vi "main.vi"() -> ()   [LabVIEW 2015]
panel:
  out "selected path":path caption="선택된 경로"
  in  "Del":bool
  in  "정지 버튼":bool
  out "원소의 인덱스":i32
  out "Right 3":cluster{"Max":u32, "Min":u32, "Delta":u32}
  out "Right 2":cluster{"Max":u32, "Min":u32, "Delta":u32}
  out "Right 1":cluster{"Max":u32, "Min":u32, "Delta":u32}
  out "Left 3":cluster{"Max":u32, "Min":u32, "Delta":u32}
  out "Left 2":cluster{"Max":u32, "Min":u32, "Delta":u32}
  out "Left 1":cluster{"Max":u32, "Min":u32, "Delta":u32}
  out "XY 그래프":cluster{"Time(s)":dbl[], "calculation":u32[]}[](graph)
  # "Chart Name"
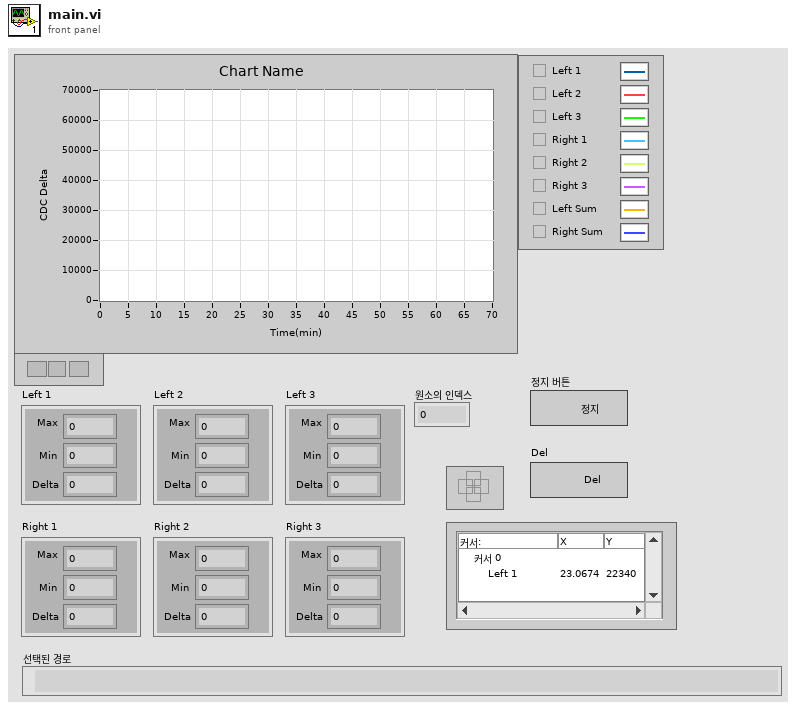
[diagram p1: front panel]
types:
  T1 = cluster{"raw data":u32[], "max":u32, "min":u32, "delta":u32, "calculation":u32[]}
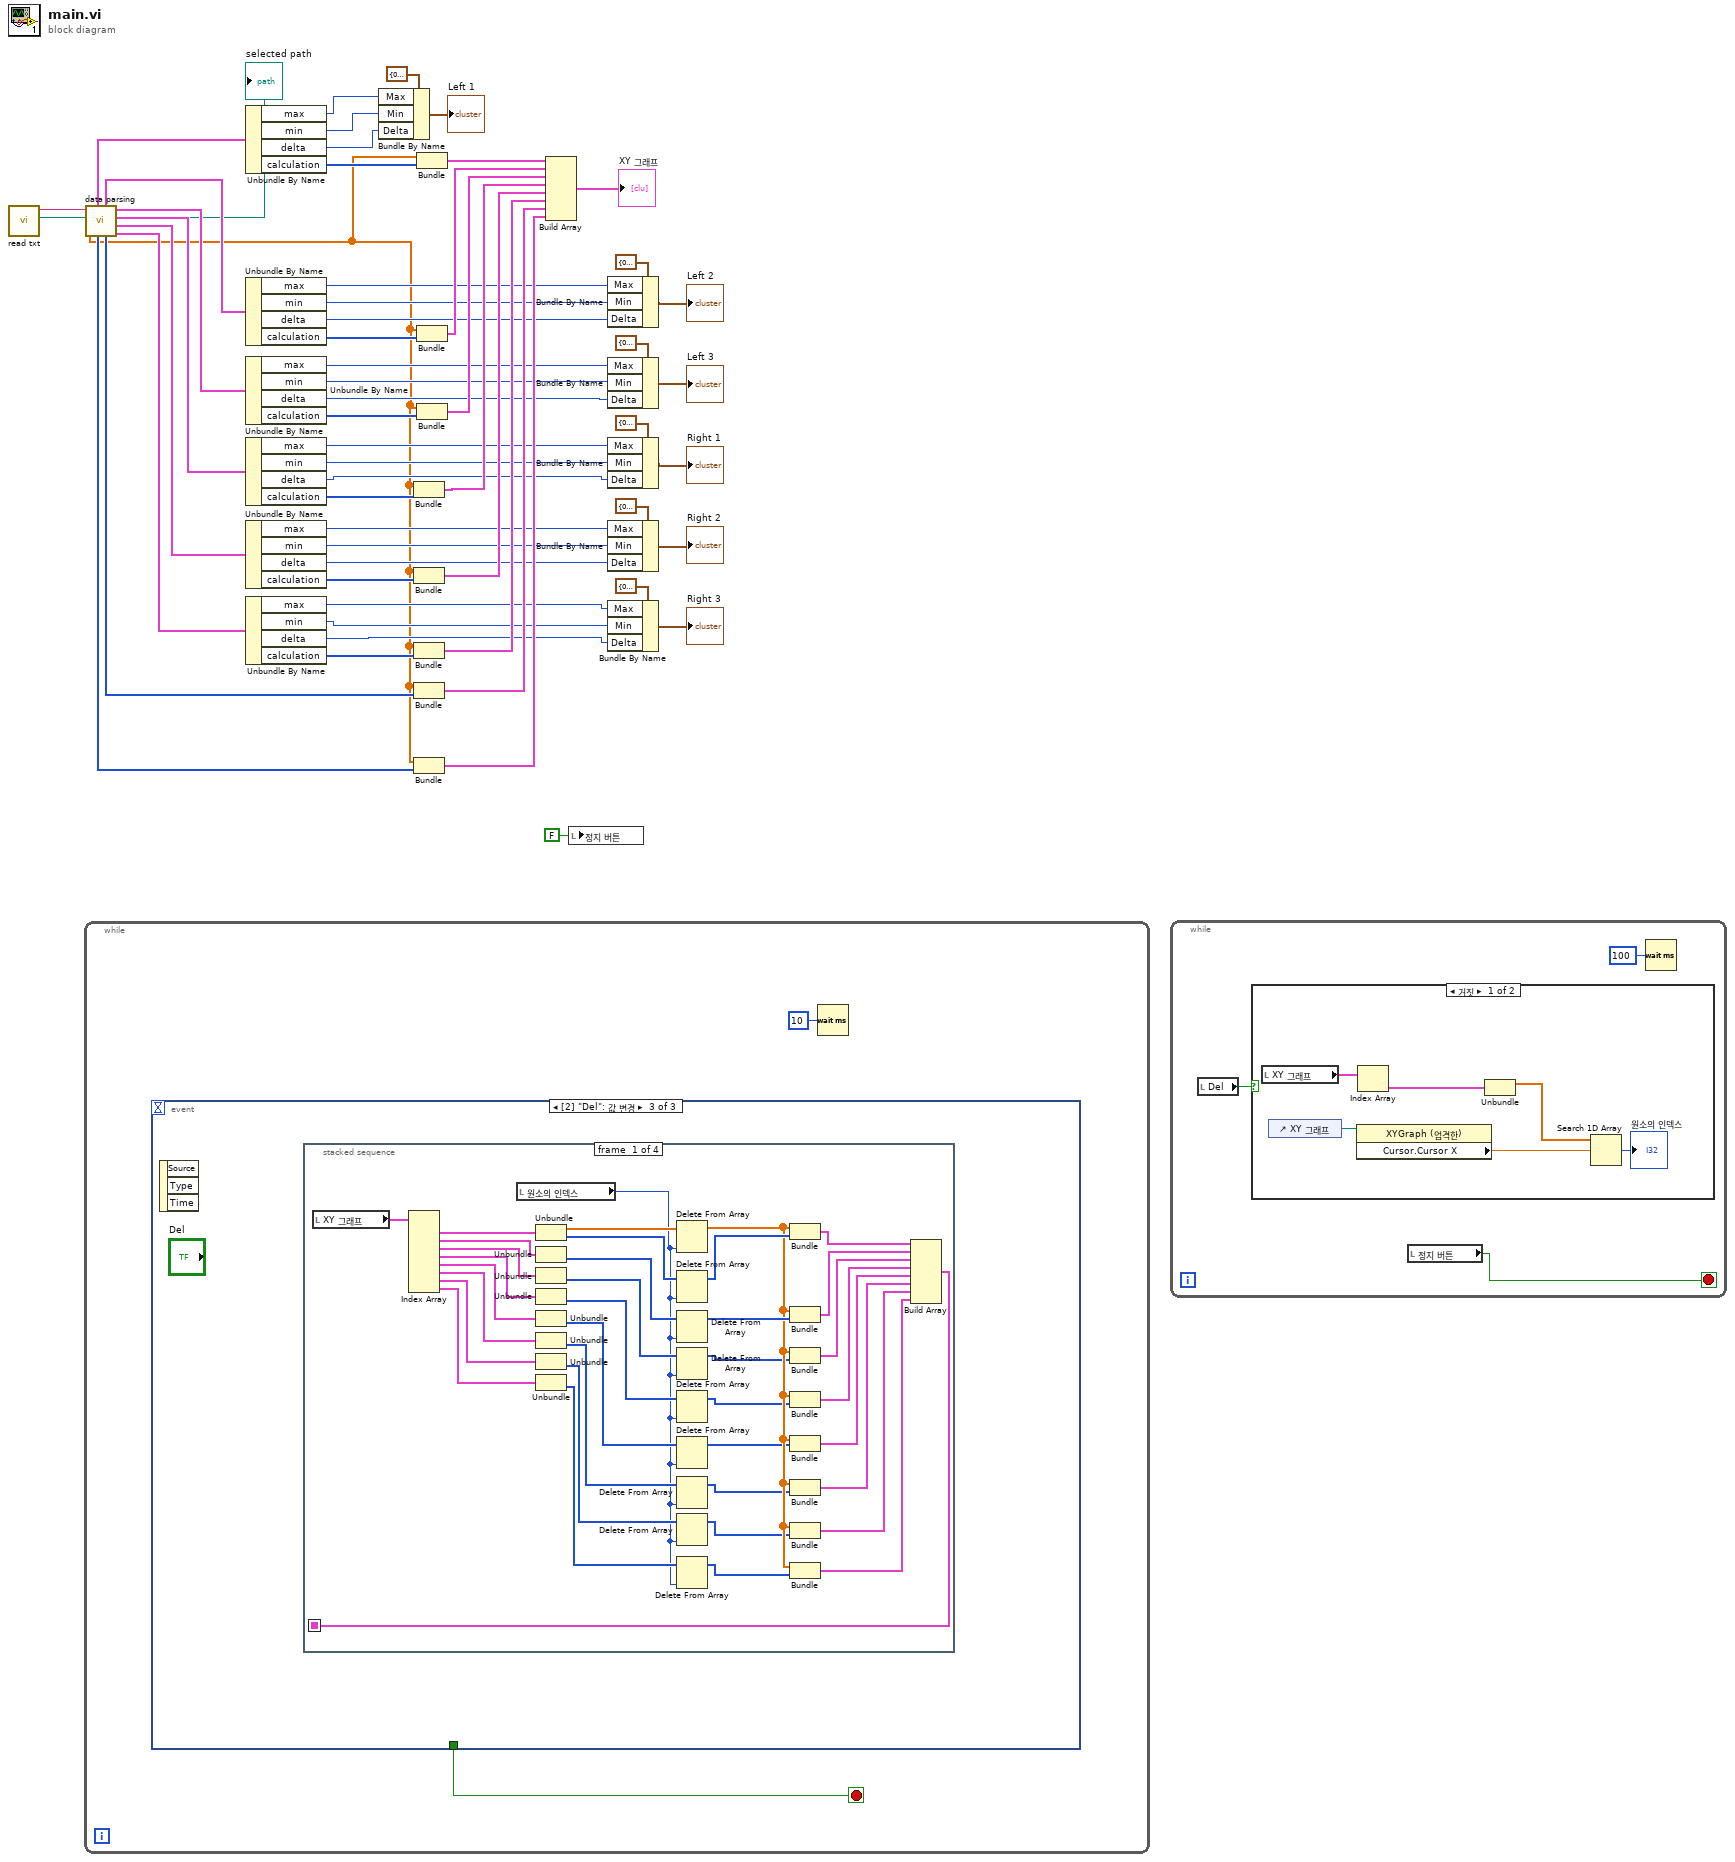
[diagram p0: block diagram]
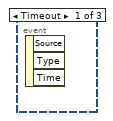
[diagram p3: hidden frame]
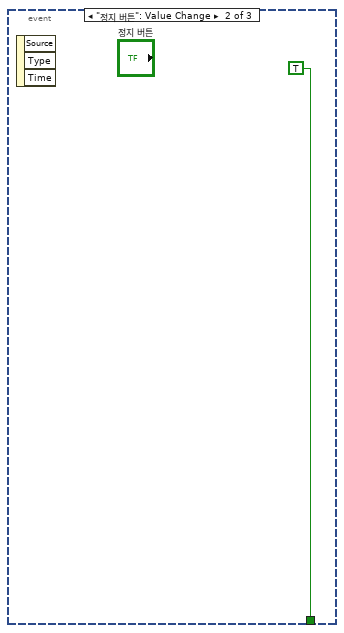
[diagram p4: hidden frame]
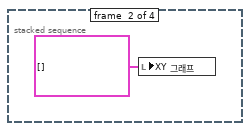
[diagram p5: hidden frame]
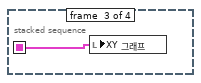
[diagram p6: hidden frame]
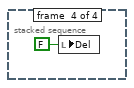
[diagram p7: hidden frame]
diagram:
  n1 = call "read txt.vi"() -> ("selected path"=→"selected path":path, "Output"=w57:string)  [unwired: 10 in]
  n2 = while {
    stop <- w59 stop-if-true
    n3 = event shown="[2] \"Del\": 값 변경" {
      selector: _ -> [_ _ _]
      dyn-events: _ -> [_ _ _]
      timeout: _ -> [_ _ _]
      tunnel: [_ TRUE _] -> w59
      event Timeout {
        n4 = event-data() -> ()  [unwired: 1 in, 3 out]
      }
      event "정지 버튼": Value Change {
        n5 = event-data() -> ()  [unwired: 1 in, 3 out]
      }
      event "Del": Value Change {
        n6 = event-data() -> ()  [unwired: 1 in, 3 out]
        n7 = stacked-sequence {
          seq-local: [w62 _ _ _] -> [_ _ w99 _]
          frame #0 {
            n8 = local read "XY 그래프"() -> (w97:cluster{"Time(s)":dbl[], "calculation":u32[]}[])
            n9 = Index Array(array=w97) -> (element #1=w96:cluster{"Time(s)":dbl[], "calculation":u32[]}, element #2=w95:cluster{"Time(s)":dbl[], "calculation":u32[]}, element #3=w94:cluster{"Time(s)":dbl[], "calculation":u32[]}, element #4=w93:cluster{"Time(s)":dbl[], "calculation":u32[]}, element #5=w92:cluster{"Time(s)":dbl[], "calculation":u32[]}, element #6=w91:cluster{"Time(s)":dbl[], "calculation":u32[]}, element #7=w90:cluster{"Time(s)":dbl[], "calculation":u32[]}, element #8=w89:cluster{"Time(s)":dbl[], "calculation":u32[]})  [unwired: 8 in]
            n10 = local read "원소의 인덱스"() -> (w61:i32)
            n11 = Unbundle(w96) -> ("Time(s)"=w88:dbl[], "calculation"=w87:u32[])
            n12 = Unbundle(w95) -> ("calculation"=w86:u32[])  [unwired: 1 out]
            n13 = Unbundle(w94) -> ("calculation"=w85:u32[])  [unwired: 1 out]
            n14 = Unbundle(w93) -> ("calculation"=w84:u32[])  [unwired: 1 out]
            n15 = Unbundle(w92) -> ("calculation"=w83:u32[])  [unwired: 1 out]
            n16 = Unbundle(w91) -> ("calculation"=w82:u32[])  [unwired: 1 out]
            n17 = Unbundle(w90) -> ("calculation"=w81:u32[])  [unwired: 1 out]
            n18 = Unbundle(w89) -> ("calculation"=w80:u32[])  [unwired: 1 out]
            n19 = Delete From Array(array=w88, index=w61) -> (array with subset deleted=w77:dbl[])  [unwired: 1 in, 1 out]
            n20 = Delete From Array(array=w87, index=w61) -> (array with subset deleted=w79:u32[])  [unwired: 1 in, 1 out]
            n21 = Delete From Array(array=w86, index=w61) -> (array with subset deleted=w78:u32[])  [unwired: 1 in, 1 out]
            n22 = Delete From Array(array=w85, index=w61) -> (array with subset deleted=w76:u32[])  [unwired: 1 in, 1 out]
            n23 = Delete From Array(array=w84, index=w61) -> (array with subset deleted=w75:u32[])  [unwired: 1 in, 1 out]
            n24 = Delete From Array(array=w83, index=w61) -> (array with subset deleted=w74:u32[])  [unwired: 1 in, 1 out]
            n25 = Delete From Array(array=w82, index=w61) -> (array with subset deleted=w73:u32[])  [unwired: 1 in, 1 out]
            n26 = Delete From Array(array=w81, index=w61) -> (array with subset deleted=w72:u32[])  [unwired: 1 in, 1 out]
            n27 = Delete From Array(array=w80, index=w61) -> (array with subset deleted=w71:u32[])  [unwired: 1 in, 1 out]
            n28 = Bundle("Time(s)"=w77, "calculation"=w79) -> (w70:cluster{"Time(s)":dbl[], "calculation":u32[]})  [unwired: 1 in]
            n29 = Bundle("Time(s)"=w77, "calculation"=w78) -> (w69:cluster{"Time(s)":dbl[], "calculation":u32[]})  [unwired: 1 in]
            n30 = Bundle("Time(s)"=w77, "calculation"=w76) -> (w68:cluster{"Time(s)":dbl[], "calculation":u32[]})  [unwired: 1 in]
            n31 = Bundle("Time(s)"=w77, "calculation"=w75) -> (w67:cluster{"Time(s)":dbl[], "calculation":u32[]})  [unwired: 1 in]
            n32 = Bundle("Time(s)"=w77, "calculation"=w74) -> (w66:cluster{"Time(s)":dbl[], "calculation":u32[]})  [unwired: 1 in]
            n33 = Bundle("Time(s)"=w77, "calculation"=w73) -> (w65:cluster{"Time(s)":dbl[], "calculation":u32[]})  [unwired: 1 in]
            n34 = Bundle("Time(s)"=w77, "calculation"=w72) -> (w64:cluster{"Time(s)":dbl[], "calculation":u32[]})  [unwired: 1 in]
            n35 = Bundle("Time(s)"=w77, "calculation"=w71) -> (w63:cluster{"Time(s)":dbl[], "calculation":u32[]})  [unwired: 1 in]
            n36 = Build Array(w70, w69, w68, w67, w66, w65, w64, w63) -> (w62:cluster{"Time(s)":dbl[], "calculation":u32[]}[])
          }
          frame #1 {
            n37 = local write "XY 그래프"(cluster{"Time(s)":dbl[], "calculation":u32[]}[] [] ("XY 그래프")) -> ()
          }
          frame #2 {
            n38 = local write "XY 그래프"(w99) -> ()
          }
          frame #3 {
            n39 = local write "Del"(FALSE ("Del")) -> ()
          }
        }
      }
    }
    n40 = Wait (ms)(milliseconds to wait=u32 10 ("대기 시간(ms)")) -> ()  [unwired: 1 out]
  }
  n41 = call "data parsing.vi"("문자열"=w57) -> ("Right 3"=w49:T1, "Right 2"=w50:T1, "Right 1"=w51:T1, "Left 3"=w52:T1, "Left_Sum"=w36:u32[], "Left 2"=w53:T1, "Right_Sum"=w37:u32[], "Left 1"=w56:T1, "Time(s)"=w3:dbl[])  [unwired: 2 in]
  n42 = Unbundle By Name(w56) -> ("max"=w31:u32, "min"=w30:u32, "delta"=w29:u32, "calculation"=w55:u32[])
  n43 = Unbundle By Name(w53) -> ("max"=w27:u32, "min"=w26:u32, "delta"=w25:u32, "calculation"=w48:u32[])
  n44 = Unbundle By Name(w52) -> ("max"=w23:u32, "min"=w22:u32, "delta"=w21:u32, "calculation"=w47:u32[])
  n45 = Unbundle By Name(w51) -> ("max"=w19:u32, "min"=w18:u32, "delta"=w17:u32, "calculation"=w46:u32[])
  n46 = Unbundle By Name(w50) -> ("max"=w11:u32, "min"=w10:u32, "delta"=w9:u32, "calculation"=w45:u32[])
  n47 = Unbundle By Name(w49) -> ("max"=w8:u32, "min"=w7:u32, "delta"=w6:u32, "calculation"=w44:u32[])
  n48 = Bundle By Name(cluster=cluster{"Max":u32, "Min":u32, "Delta":u32} {"Max"=0, "Min"=0, "Delta"=0} ("Left 1"), "Max"=w31, "Min"=w30, "Delta"=w29) -> (→"Left 1":cluster{"Max":u32, "Min":u32, "Delta":u32})
  n49 = Bundle("Time(s)"=w3, "calculation"=w46) -> (w41:cluster{"Time(s)":dbl[], "calculation":u32[]})  [unwired: 1 in]
  n50 = Bundle("Time(s)"=w3, "calculation"=w45) -> (w40:cluster{"Time(s)":dbl[], "calculation":u32[]})  [unwired: 1 in]
  n51 = Bundle("Time(s)"=w3, "calculation"=w44) -> (w38:cluster{"Time(s)":dbl[], "calculation":u32[]})  [unwired: 1 in]
  n52 = Bundle("Time(s)"=w3, "Left_Sum"=w36) -> (w35:cluster{"Time(s)":dbl[], "Left_Sum":u32[]})  [unwired: 1 in]
  n53 = Bundle("Time(s)"=w3, "Right_Sum"=w37) -> (w34:cluster{"Time(s)":dbl[], "Right_Sum":u32[]})  [unwired: 1 in]
  n54 = Bundle("Time(s)"=w3, "calculation"=w55) -> (w54:cluster{"Time(s)":dbl[], "calculation":u32[]})  [unwired: 1 in]
  n55 = Bundle("Time(s)"=w3, "calculation"=w48) -> (w43:cluster{"Time(s)":dbl[], "calculation":u32[]})  [unwired: 1 in]
  n56 = Bundle("Time(s)"=w3, "calculation"=w47) -> (w42:cluster{"Time(s)":dbl[], "calculation":u32[]})  [unwired: 1 in]
  n57 = Build Array(w54, w43, w42, w41, w40, w38, w35, w34) -> (→"XY 그래프":cluster{"Time(s)":dbl[], "Right_Sum":u32[]}[])
  n58 = local write "정지 버튼"(FALSE ("정지 버튼")) -> ()
  n59 = Bundle By Name(cluster=cluster{"Max":u32, "Min":u32, "Delta":u32} {"Max"=0, "Min"=0, "Delta"=0} ("Left 1"), "Max"=w27, "Min"=w26, "Delta"=w25) -> (→"Left 2":cluster{"Max":u32, "Min":u32, "Delta":u32})
  n60 = Bundle By Name(cluster=cluster{"Max":u32, "Min":u32, "Delta":u32} {"Max"=0, "Min"=0, "Delta"=0} ("Left 1"), "Max"=w23, "Min"=w22, "Delta"=w21) -> (→"Left 3":cluster{"Max":u32, "Min":u32, "Delta":u32})
  n61 = Bundle By Name(cluster=cluster{"Max":u32, "Min":u32, "Delta":u32} {"Max"=0, "Min"=0, "Delta"=0} ("Left 1"), "Max"=w19, "Min"=w18, "Delta"=w17) -> (→"Right 1":cluster{"Max":u32, "Min":u32, "Delta":u32})
  n62 = Bundle By Name(cluster=cluster{"Max":u32, "Min":u32, "Delta":u32} {"Max"=0, "Min"=0, "Delta"=0} ("Left 1"), "Max"=w11, "Min"=w10, "Delta"=w9) -> (→"Right 2":cluster{"Max":u32, "Min":u32, "Delta":u32})
  n63 = Bundle By Name(cluster=cluster{"Max":u32, "Min":u32, "Delta":u32} {"Max"=0, "Min"=0, "Delta"=0} ("Left 1"), "Max"=w8, "Min"=w7, "Delta"=w6) -> (→"Right 3":cluster{"Max":u32, "Min":u32, "Delta":u32})
  n64 = while {
    stop <- w103 stop-if-true
    n65 = local read "Del"() -> (w101:bool)
    n66 = case shown="거짓" w101 {
      frame False {
        n67 = local read "XY 그래프"() -> (w107:cluster{"Time(s)":dbl[], "calculation":u32[]}[])
        n68 = control-ref of="XY 그래프"() -> (w105:refnum<vi>)
        n69 = property class="XYGraph (엄격한)"(reference=w105) -> ("Cursor.Cursor X"=w106:dbl)  [unwired: 1 in, 2 out]
        n70 = Index Array(array=w107) -> (element=w108:cluster{"Time(s)":dbl[], "calculation":u32[]})  [unwired: 1 in]
        n71 = Unbundle(w108) -> ("Time(s)"=w109:dbl[])  [unwired: 1 out]
        n72 = Search 1D Array(1D array=w109, element=w106) -> (index of element=→"원소의 인덱스":i32)  [unwired: 1 in]
      }
      frame True {
      }
    }
    n73 = local read "정지 버튼"() -> (w103:bool)
    n74 = Wait (ms)(milliseconds to wait=u32 100 ("대기 시간(ms)")) -> ()  [unwired: 1 out]
  }
